vi "picoquant_acquire_stream.vi"(8 "error in (no error)":errorcluster, 10 "picoquant_panel":refnum<class "panel.lvclass">, 11 "picoquant_generic in":refnum<class "picoquant_generic.lvclass">) -> (0 "error out":errorcluster, 2 "panel out":refnum<class "panel.lvclass">, 3 "picoquant_generic out":refnum<class "picoquant_generic.lvclass">)   [LabVIEW 2015, in "picoquant_generic.lvclass"]
uses:
  picoquant_generic.lvclass
  UI/panel_class/panel.lvclass
  UI/panel_class/panel.lvclass/panel.ctl
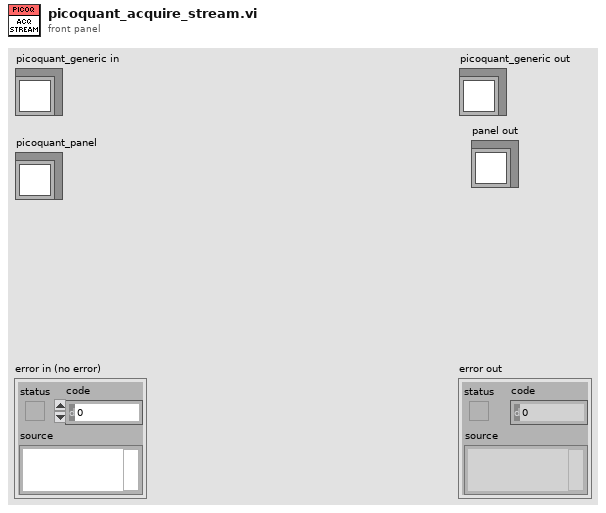
[diagram p1: front panel]
types:
  T1 = typedef "ui_user_events.ctl" = cluster{"update_xy_graph":refnum<user-event>, "update_graph":refnum<user-event>, "update_chart":refnum<user-event>, "update_map":refnum<user-event>, "event_loop_stop":refnum<user-event>, "keep_map":refnum<user-event>}
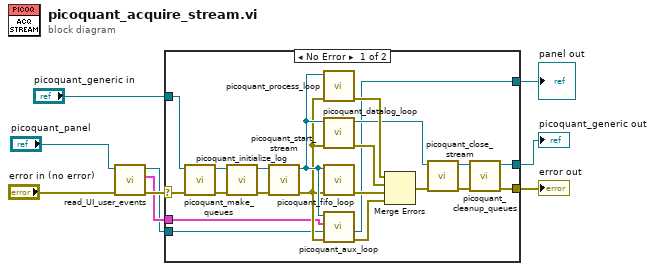
[diagram p0: block diagram]
diagram:
  n1 = call "read_UI_user_events.vi"("error in (no error)"="error in (no error)", "panel in"="picoquant_panel") -> ("error out"=w4:errorcluster, "ui_user_events"=w3:T1, "panel out"=w1:refnum<class "panel.lvclass">)  [unwired: 7 in]
  n2 = case shown="No Error" w4 {
    selector: w4 -> [w22 w33]
    tunnel: [w18 w33] -> w9
    tunnel: [w17 w32] -> w7
    tunnel: "picoquant_generic in" -> [w21 w32]
    tunnel: w3 -> [w16 _]
    tunnel: [w10 w31] -> w2
    tunnel: w1 -> [w11 w31]
    frame No Error {
      n3 = call "picoquant_make_queues.vi"("error in (no error)"=w22, "picoquant_generic in"=w21) -> ("error out"=w24:errorcluster, "picoquant_generic out"=w23:refnum<class "picoquant_generic.lvclass">)  [unwired: 8 in]
      n4 = call-dynamic "picoquant_initialize_log.vi"("error in (no error)"=w24, "picoquant_generic in"=w23) -> ("error out"=w19:errorcluster, "picoquant_generic out"=w20:refnum<class "picoquant_generic.lvclass">)  [unwired: 8 in]
      n5 = call-dynamic "picoquant_start_stream.vi"("error in (no error)"=w19, "picoquant_generic in"=w20) -> ("error out"=w29:errorcluster, "picoquant_generic out"=w30:refnum<class "picoquant_generic.lvclass">)  [unwired: 8 in]
      n6 = call "picoquant_process_loop.vi"("error in (no error)"=w29, "picoquant_generic in"=w30) -> ("error out"=w28:errorcluster)  [unwired: 8 in, 1 out]
      n7 = call "picoquant_datalog_loop.vi"("error in (no error)"=w29, "picoquant_generic in"=w30) -> ("error out"=w27:errorcluster, "picoquant_generic out"=w14:refnum<class "picoquant_generic.lvclass">)  [unwired: 8 in]
      n8 = call "picoquant_fifo_loop.vi"("error in (no error)"=w29, "picoquant_generic in"=w30) -> ("error out"=w26:errorcluster)  [unwired: 8 in, 1 out]
      n9 = call "picoquant_aux_loop.vi"("error in (no error)"=w29, "panel_in"=w11, "ui_user_events"=w16, "picoquant_generic in"=w30) -> ("error out"=w25:errorcluster, "panel_out"=w10:refnum<class "panel.lvclass">)  [unwired: 5 in, 1 out]
      n10 = Merge Errors(w28, w27, w26, w25) -> (w15:errorcluster)
      n11 = call-dynamic "picoquant_close_stream.vi"("error in (no error)"=w15, "picoquant_generic in"=w14) -> ("error out"=w12:errorcluster, "picoquant_generic out"=w13:refnum<class "picoquant_generic.lvclass">)  [unwired: 8 in]
      n12 = call "picoquant_cleanup_queues.vi"("error in (no error)"=w12, "picoquant_generic in"=w13) -> ("error out"=w18:errorcluster, "picoquant_generic out"=w17:refnum<class "picoquant_generic.lvclass">)  [unwired: 8 in]
    }
    frame Error {
    }
  }
  "error out" <- w9
  "picoquant_generic out" <- w7
  "panel out" <- w2
